vi "file test.vi"() -> ()   [LabVIEW 2013, in "TEC tests.lvlib"]
uses:
  TEC tests.lvlib
  <vilib>/NI/Tag Bus Module Framework/module configuration/TBM module configuration.lvclass
  <vilib>/NI/Configuration Framework/class discovery singleton/class discovery singleton methods.ctl
  execution/TEC runtime.lvclass
  configuration/TEC configuration.lvclass
  configuration/TEC configuration.lvclass/TEC configuration.ctl
  <vilib>/NI/Tag Bus/table/data polymorphs/write one/write Double.vi
  <vilib>/NI/Tag Bus/table/data polymorphs/read one/read Double.vi
  configuration/Write receive on port.vi
  configuration/Write send from port.vi
  configuration/Write send to address.vi
  configuration/Write send to port.vi
  <vilib>/NI/Configuration Framework/tree serializer/NISE_CEF_TreeSerializer.lvlib
  <vilib>/NI/Tag Bus Data Framework/Framework Configuration Classes/flattened data interface/PL_Serialization Interface.lvlib
  <vilib>/NI/Configuration Framework/class discovery singleton/class discovery singleton.lvlib
  <vilib>/NI/Tag Bus/table/data table.lvlib
  <vilib>/ptbypt/NI_PtbyPt.lvlib
panel:
  out "final":errorcluster
  in  "stop":bool
  in  "value tx":dbl
  out "value rx":dbl
  out "timeout count":u16
  out "duration":dbl
  in  "millisecond multiple":u32=100
  out "duration avg":dbl
  out "init err":errorcluster
  in  "target":i32
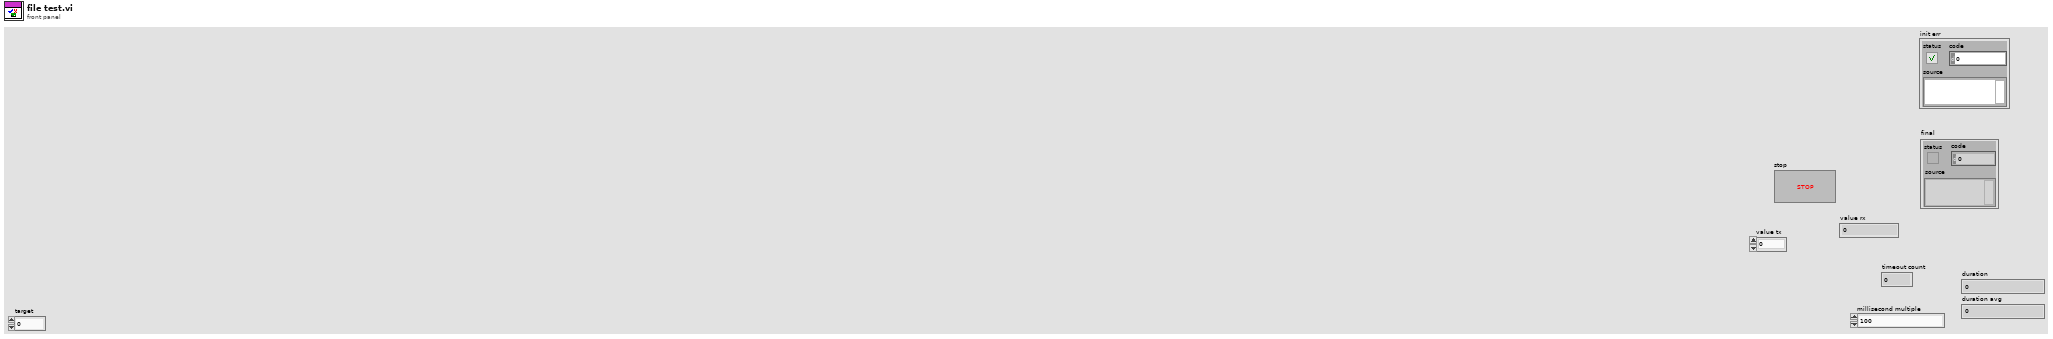
[diagram p1: front panel]
types:
  T1 = typedef "class discovery singleton.lvlib/class discovery singleton methods.ctl" = enum16{"add search paths", "load class by name", "list available classes", "get class path"}
  T2 = typedef "NISE_CEF_TreeSerializer.lvlib/base file format.ctl" = cluster{"version":string, "data":string}
  T3 = typedef "NISE_CEF_TreeSerializer.lvlib/flat hierarchy.ctl" = cluster{"hierarchy structure":T4, "instance data":T6[]}
  T4 = typedef "NISE_CEF_TreeSerializer.lvlib/full hierarchy.ctl" = cluster{"root":string, "hierarchy":T5[]}
  T5 = typedef "NISE_CEF_TreeSerializer.lvlib/hierarchy element.ctl" = cluster{"current node":string, "children":string[]}
  T6 = typedef "NISE_CEF_TreeSerializer.lvlib/instance data.ctl" = cluster{"ID":string, "Alias":string, "class":string, "version":string, "data":string}
  T7 = typedef "NISE_CEF_TreeSerializer.lvlib/memory hierarchy.ctl" = cluster{"hierarchy structure":T4, "instance data":refnum<class "NISE_CEF_serializable configuration.lvclass">[]}
  T8 = typedef "TBM channel.lvclass/data tables.ctl" = cluster{"input data":T9, "processing parameter":T9, "processing result":T9, "output data":T9}
  T9 = typedef "tag bus.lvlib/dictionary table pair.ctl" = cluster{"data dictionary":refnum<class "data dictionary.lvclass">, "data table":T10}
  T10 = typedef "tag bus.lvlib/data table.lvlib/data table.ctl" = cluster{"Double":dbl[], "Single":sgl[], "I64":i64[], "I32":i32[], "I16":i16[], "I8":i8[], "U64":u64[], "U32":u32[], "U16":u16[], "U8":u8[], "Boolean":bool[], "String":string[], "Array of Double":cluster{"DBL Array":dbl[]}[], "Array of Single":cluster{"SGL Array":sgl[]}[], "Array of I64":cluster{"I64 Array":i64[]}[], "Array of I32":cluster{"I32 Array":i32[]}[], "Array of I16":cluster{"I16 Array":i16[]}[], "Array of I8":cluster{"I8 Array":i8[]}[], "Array of U64":cluster{"U64 Array":u64[]}[], "Array of U32":cluster{"U32 Array":u32[]}[], "Array of U16":cluster{"U16 Array":u16[]}[], "Array of U8":cluster{"U8 Array":u8[]}[], "Array of Boolean":cluster{"Boolean Array":bool[]}[], "Array of String":cluster{"String Array":string[]}[]}
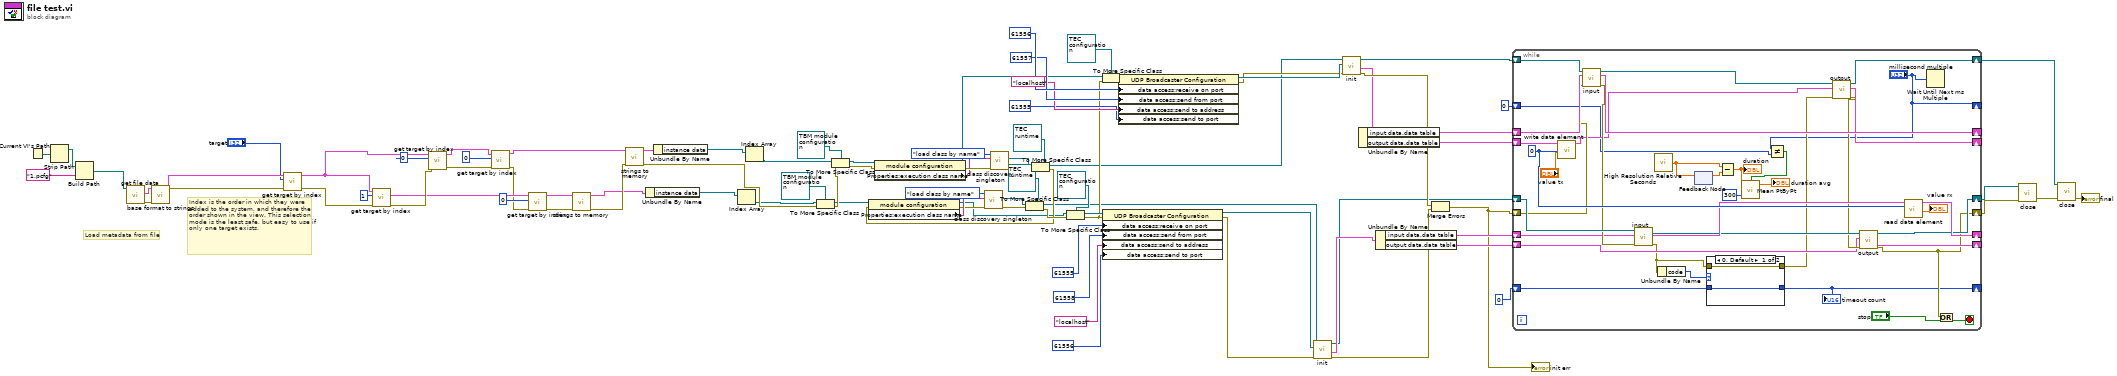
[diagram p0: block diagram]
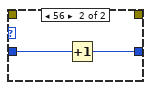
[diagram p2: hidden frame]
diagram:
  # "Index is the order in which they were added to the system, and therefore the order shown in the view. This selection mode is the least safe, but easy to use if only one target exists."
  # "Load metadata from file"
  n1 = Current VI's Path() -> (path=w87:path)
  n2 = Strip Path(path=w87) -> (stripped path=w86:path)  [unwired: 1 out]
  n3 = Build Path(base path=w86, name or relative path="1.pcfg") -> (appended path=w84:path)
  n4 = call <vilib>:"get file data.vi"("Path"=w84) -> ("error out"=w91:errorcluster, "format"=w90:T2)  [unwired: 9 in]
  n5 = call <vilib>:"base format to strings.vi"("error in"=w91, "format"=w90) -> ("error out"=w89:errorcluster, "data"=w88:T3)  [unwired: 8 in]
  n6 = call <vilib>:"get target by index.vi"("error in"=w89, "index"="target", "system hierarchy"=w88) -> ("error out"=w80:errorcluster, "target hierarchy"=w83:T3)  [unwired: 7 in]
  n7 = call <vilib>:"get target by index.vi"("error in"=w80, "index"=1, "system hierarchy"=w83) -> ("error out"=w79:errorcluster, "target hierarchy"=w74:T3)  [unwired: 7 in]
  n8 = call <vilib>:"get target by index.vi"("error in"=w79, "index"=0, "system hierarchy"=w83) -> ("error out"=w77:errorcluster, "target hierarchy"=w78:T3)  [unwired: 7 in]
  n9 = call <vilib>:"get target by index.vi"("error in"=w77, "index"=0, "system hierarchy"=w78) -> ("error out"=w73:errorcluster, "target hierarchy"=w72:T3)  [unwired: 7 in]
  n10 = call <vilib>:"get target by index.vi"("error in"=w73, "index"=0, "system hierarchy"=w74) -> ("error out"=w70:errorcluster, "target hierarchy"=w69:T3)  [unwired: 7 in]
  n11 = call <vilib>:"strings to memory.vi"("error in"=w70, "1.0.0"=w69) -> ("error out"=w71:errorcluster, "memory hierarchy"=w65:T7)  [unwired: 8 in]
  n12 = call <vilib>:"strings to memory.vi"("error in"=w71, "1.0.0"=w72) -> ("error out"=w62:errorcluster, "memory hierarchy"=w68:T7)  [unwired: 8 in]
  n13 = Unbundle By Name(w65) -> ("instance data"=w66:refnum<class "NISE_CEF_serializable configuration.lvclass">[])
  n14 = Unbundle By Name(w68) -> ("instance data"=w67:refnum<class "NISE_CEF_serializable configuration.lvclass">[])
  n15 = Index Array(array=w66) -> (element=w59:refnum<class "NISE_CEF_serializable configuration.lvclass">)  [unwired: 1 in]
  n16 = Index Array(array=w67) -> (element=w63:refnum<class "NISE_CEF_serializable configuration.lvclass">)  [unwired: 1 in]
  n17 = To More Specific Class(target class=refnum<class "TBM module configuration.lvclass"> refnum ("module configuration"), reference=w59, error in=w62) -> (specific class reference=w43:refnum<class "TBM module configuration.lvclass">, error out=w61:errorcluster)
  n18 = To More Specific Class(target class=refnum<class "TBM module configuration.lvclass"> refnum ("module configuration"), reference=w63, error in=w61) -> (specific class reference=w57:refnum<class "TBM module configuration.lvclass">, error out=w56:errorcluster)
  n19 = property class="module configuration"(reference=w57, error in=w56) -> (reference out=w29:refnum<class "TBM module configuration.lvclass">, error out=w55:errorcluster, "Properties:execution class name"=w54:string)
  n20 = call <vilib>:"class discovery singleton.vi"("error in"=w55, "Class Name"=w54, "method"=class_discovery_singleton_methods."load class by name") -> ("error out"=w52:errorcluster, "LabVIEW Object"=w51:refnum<class>)  [unwired: 5 in, 2 out]
  n21 = To More Specific Class(target class=refnum<class "TEC runtime.lvclass"> refnum ("UDP Broadcaster Runtime"), reference=w51, error in=w52) -> (specific class reference=w4:refnum<class "TEC runtime.lvclass">, error out=w33:errorcluster)
  n22 = property class="module configuration"(reference=w43, error in=w33) -> (reference out=w32:refnum<class "TBM module configuration.lvclass">, error out=w44:errorcluster, "Properties:execution class name"=w45:string)
  n23 = call <vilib>:"class discovery singleton.vi"("error in"=w44, "Class Name"=w45, "method"=class_discovery_singleton_methods."load class by name") -> ("error out"=w47:errorcluster, "LabVIEW Object"=w48:refnum<class>)  [unwired: 5 in, 2 out]
  n24 = To More Specific Class(target class=refnum<class "TEC runtime.lvclass"> refnum ("UDP Broadcaster Runtime"), reference=w48, error in=w47) -> (specific class reference=w1:refnum<class "TEC runtime.lvclass">, error out=w34:errorcluster)
  n25 = To More Specific Class(target class=refnum<class "TEC configuration.lvclass"> refnum ("UDP Broadcaster Configuration"), reference=w32, error in=w34) -> (specific class reference=w31:refnum<class "TEC configuration.lvclass">, error out=w27:errorcluster)
  n26 = To More Specific Class(target class=refnum<class "TEC configuration.lvclass"> refnum ("UDP Broadcaster Configuration"), reference=w29, error in=w27) -> (specific class reference=w30:refnum<class "TEC configuration.lvclass">, error out=w28:errorcluster)
  n27 = property class="UDP Broadcaster Configuration"(reference=w31, error in=w27, "data access:receive on port"=u16 61555 ("send from port"), "data access:send from port"=u16 61558 ("send to port"), "data access:send to address"="localhost" ("send to address"), "data access:send to port"=u16 61556 ("receive on port")) -> (reference out=w3:refnum<class "TEC configuration.lvclass">, error out=w2:errorcluster)
  n28 = property class="UDP Broadcaster Configuration"(reference=w30, error in=w28, "data access:receive on port"=u16 61556 ("send from port"), "data access:send from port"=u16 61557 ("send to port"), "data access:send to address"="localhost" ("send to address"), "data access:send to port"=u16 61555 ("receive on port")) -> (reference out=w6:refnum<class "TEC configuration.lvclass">, error out=w5:errorcluster)
  n29 = call-dynamic "init.vi"("error in"=w2, "TBM module configuration in"=w3, "TEC runtime in"=w1) -> ("error out"=w23:errorcluster, "data allocations"=w21:T8, "TEC runtime out"=w15:refnum<class "TEC runtime.lvclass">)  [unwired: 5 in, 1 out]
  n30 = call-dynamic "init.vi"("error in"=w5, "TBM module configuration in"=w6, "TEC runtime in"=w4) -> ("error out"=w24:errorcluster, "data allocations"=w22:T8, "TEC runtime out"=w16:refnum<class "TEC runtime.lvclass">)  [unwired: 5 in, 1 out]
  n31 = Unbundle By Name(w22) -> ("input data.data table"=w18:T10, "output data.data table"=w17:T10)
  n32 = Unbundle By Name(w21) -> ("input data.data table"=w20:T10, "output data.data table"=w19:T10)
  n33 = Merge Errors(w24, w23) -> (w14:errorcluster)
  "init err" <- w14
  n34 = while {
    shift-right: [w125] -> _
    shift-left: w20 -> [w116]
    shift-right: [w108] -> _
    shift-left: w19 -> [w105]
    shift-right: [w111] -> _
    shift-left: w17 -> [w127]
    shift-right: [w120] -> _
    shift-left: w18 -> [w121]
    shift-right: [w113] -> w10
    shift-left: w16 -> [w122]
    shift-right: [w109] -> w9
    shift-left: w15 -> [w119]
    shift-right: [w106] -> w13
    shift-left: w14 -> [w118]
    shift-right: [w101] -> _
    shift-left: u16 0 ("Numeric") -> [w100]
    shift-right: ["millisecond multiple"] -> _
    shift-left: u32 0 ("millisecond multiple") -> [w94]
    stop <- w128 stop-if-true
    w123 = 0 ("index")
    n35 = call-poly <vilib>:"write data element.vi"("value"="value tx", "index"=w123, "data table in"=w127) -> ("data table out"=w112:T10)  [unwired: 8 in]
    n36 = call-dynamic "input.vi"("error in"=w118, "data table in"=w121, "TEC runtime in"=w122) -> ("error out"=w117:errorcluster, "data table out"=w120:T10, "TEC runtime out"=w114:refnum<class "TEC runtime.lvclass">)  [unwired: 6 in]
    n37 = call-dynamic "input.vi"("error in"=w117, "data table in"=w116, "TEC runtime in"=w119) -> ("error out"=w103:errorcluster, "data table out"=w115:T10, "TEC runtime out"=w110:refnum<class "TEC runtime.lvclass">)  [unwired: 6 in]
    n38 = call <vilib>:"High Resolution Relative Seconds.vi"() -> ("relative seconds"=w98:dbl)
    n39 = Unbundle By Name(w103) -> ("code"=w104:i32)
    n40 = feedback-in #1(w98) -> ()
    n41 = feedback #1() -> (w99:dbl)  [unwired: 1 in]
    n42 = case shown="0, Default" w104 {
      tunnel: w103 -> [w131 _]
      tunnel: [w131 _] -> w102
      tunnel: [w130 w133] -> w101
      tunnel: w100 -> [w130 w132]
      frame 0, Default {
      }
      frame 56 {
        n43 = Increment(x=w132) -> (x+1=w133:u16)
      }
    }
    "timeout count" <- w101
    n44 = Subtract(x=w98, y=w99) -> (x-y=w97:dbl)
    "duration" <- w97
    n45 = Not Equal?(x="millisecond multiple", y=w94) -> (x != y?=w93:bool)
    n46 = call <vilib>:"Mean PtByPt.vi"("x"=w97, "sample length"=300, "initialize"=w93) -> ("mean"=→"duration avg":dbl)  [unwired: 1 in, 1 out]
    n47 = call-dynamic "output.vi"("error in"=w102, "data table in"=w112, "TEC runtime in"=w114) -> ("error out"=w107:errorcluster, "data table out"=w111:T10, "TEC runtime out"=w113:refnum<class "TEC runtime.lvclass">)  [unwired: 6 in]
    n48 = call-dynamic "output.vi"("error in"=w107, "data table in"=w105, "TEC runtime in"=w110) -> ("error out"=w106:errorcluster, "data table out"=w108:T10, "TEC runtime out"=w109:refnum<class "TEC runtime.lvclass">)  [unwired: 6 in]
    n49 = call-poly <vilib>:"read data element.vi"("index"=w123, "data table in"=w115) -> ("value"=→"value rx":dbl, "data table out"=w125:T10)  [unwired: 8 in]
    n50 = Wait Until Next ms Multiple(millisecond multiple="millisecond multiple") -> ()  [unwired: 1 out]
    n51 = Or(x=w106, y="stop") -> (x .or. y?=w128:bool)
  }
  n52 = call-dynamic "close.vi"("error in"=w13, "TEC runtime in"=w9) -> ("error out"=w12:errorcluster)  [unwired: 9 in]
  n53 = call-dynamic "close.vi"("error in"=w12, "TEC runtime in"=w10) -> ("error out"=→"final":errorcluster)  [unwired: 9 in]
